vi "Stop Measurements.vi"(8 "error in (no error)":errorcluster, 11 "Monitor Controller in":refnum<class "Monitor Controller.lvclass">) -> (0 "error out":errorcluster, 3 "Monitor Controller out":refnum<class "Monitor Controller.lvclass">)   [LabVIEW 2016, in "Monitor Controller.lvclass"]
uses:
  Monitor Controller.lvclass
  C:/github/LabActor/Worker/Worker.lvclass
  C:/Program Files/National Instruments/LabVIEW 2016/vi.lib/ActorFramework/Actor/Actor.lvclass
  C:/github/LabActor/Template Module/Template Module.lvclass
  Worker/Worker.lvclass/Worker.ctl
  <vilib>/ActorFramework/Actor/Actor.lvclass/Actor.ctl
  Update Monitor State Msg/Update Monitor State Msg.lvclass/Update Monitor State Msg.ctl
  <vilib>/ActorFramework/Message Enqueuer/Message Enqueuer.lvclass/Message Enqueuer.ctl
  Template Module/Template Module.lvclass/Template Module.ctl
  Template Module/Read tdms stream.vi
  Template Module/Read State.vi
  <vilib>/ActorFramework/Message Enqueuer/Enqueue.vi
  Update Monitor State Msg/Update Monitor State Msg.lvclass
  C:/Program Files/National Instruments/LabVIEW 2016/vi.lib/ActorFramework/Message/Message.lvclass
  <vilib>/ActorFramework/Message Priority Queue/Priority Enqueue.vi
  Process Controller/Process Controller.lvclass
  <vilib>/ActorFramework/Actor/Actor.lvclass
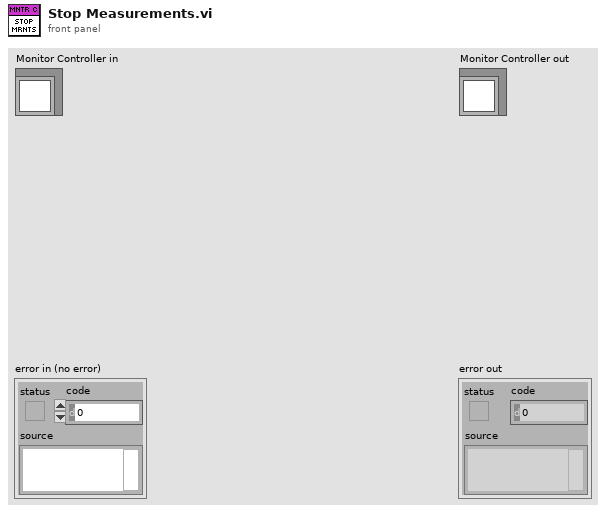
[diagram p1: front panel]
types:
  T1 = typedef "Worker State.ctl" = enum16{"Idle", "Starting", "Working", "Stopping"}
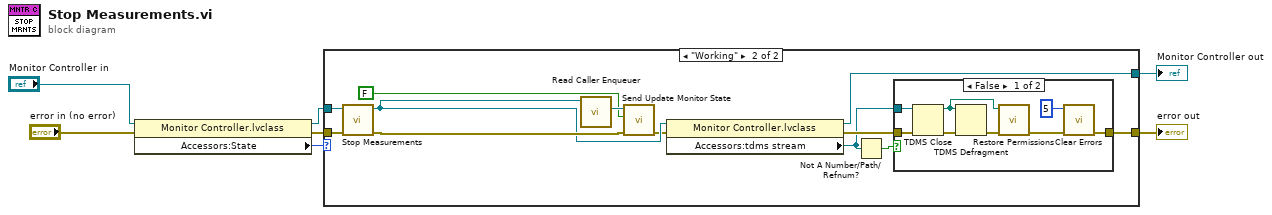
[diagram p0: block diagram]
diagram:
  n1 = property class="Monitor Controller.lvclass"(reference="Monitor Controller in", error in="error in (no error)") -> (reference out=w3:refnum<class "Monitor Controller.lvclass">, error out=w2:errorcluster, "Accessors:State"=w5:T1)
  n2 = case shown="\"Working\"" w5 {
    tunnel: w2 -> [w8 w21]
    tunnel: w3 -> [w9 w20]
    tunnel: [w9 w11] -> w7
    tunnel: [w8 w10] -> w6
    frame "Idle", Default {
    }
    frame "Working" {
      n3 = call-parent "Stop Measurements.vi"("error in (no error)"=w21, "Measure Controller in"=w20) -> ("error out"=w16:errorcluster, "Measure Controller out"=w13:refnum<class "Monitor Controller.lvclass">)  [unwired: 8 in]
      n4 = call <vilib>:"Read Caller Enqueuer.vi"("Actor"=w13) -> ("Caller Enqueuer"=w18:refnum<class "Message Enqueuer.lvclass">)  [unwired: 10 in]
      n5 = call "Send Update Monitor State.vi"("error in (no error)"=w16, "Monitor Running"=FALSE, "Message Enqueuer"=w18) -> ("error out"=w12:errorcluster)  [unwired: 7 in, 1 out]
      n6 = property class="Monitor Controller.lvclass"(reference=w13, error in=w12) -> (reference out=w11:refnum<class "Monitor Controller.lvclass">, error out=w19:errorcluster, "Accessors:tdms stream"=w15:refnum<k34>)
      n7 = Not A Number/Path/Refnum?(number/path/refnum=w15) -> (NaN/Path/Refnum?=w14:bool)
      n8 = case shown="False" w14 {
        tunnel: w19 -> [w29 w30]
        tunnel: [w27 w30] -> w10
        tunnel: w15 -> [w25 _]
        frame False {
          n9 = TDMS Close(8:w29, 11:w25) -> (0:w28:errorcluster, 3:w22:path)
          n10 = TDMS Defragment(4:w28, 7:w22) -> (0:w24:errorcluster)
          n11 = call "Restore Permissions.vi"("Error In"=w24, "File Path"=w22) -> ("Error Out"=w23:errorcluster)  [unwired: 8 in, 1 out]
          n12 = call <vilib>:"Clear Errors.vi"("error in (no error)"=w23, "specific error code to clear (0: all)"=5) -> ("error out"=w27:errorcluster)  [unwired: 4 in, 1 out]
        }
        frame True {
        }
      }
    }
  }
  "error out" <- w6
  "Monitor Controller out" <- w7
